vi "Halfband Filter.vi"() -> ()   [LabVIEW 2023]
doc: "Demonstrates how to use the DFD Halfband Design VI to design a halfband finite impulse response (FIR) filter.\n\nComplete the following steps to use this VI.\n1) Run the VI.\n2) Change the specifications and run this VI again.\n3) Observe the Coefficients and Magnitude Response graphs. Notice that the filter coefficients equal zero every other coefficient except for the middle coefficient."
uses:
  <vilib>/addons/Digital Filter Design/_Objects.llb/DFD Multirate Filtering Mode.ctl
  <vilib>/addons/Digital Filter Design/NI_DigFilterLicensed.lvlib
panel:
  out "Error Message":string
  in  "Method":u16(ring)=3 items=["Kaiser Window", "Dolph-Chebyshev Window", "Equi-Ripple", "Positive Equi-Ripple", "Max Flat"]
  in  "Filter Type":enum16{"Lowpass", "Highpass"}(ring)
  in  "Roll Off":dbl=0.1
  out "Magnitude Response":cluster{"f0":dbl, "df":dbl, "values":dbl[]}[](graph)
  out "Coefficients":dbl[](graph)
  in  "Stopband Attenuation [dB]":dbl=40.0 format="%.2f"
  # "Select Help>>Show Context Help and move the cursor over the VI icon for more information."
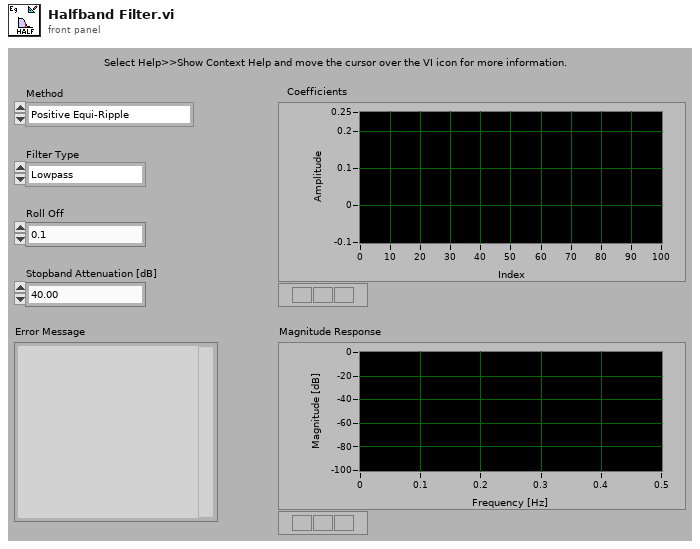
[diagram p1: front panel]
types:
  T1 = typedef "NI_DigFilterLicensed.lvlib/DFD Multirate Filtering Mode.ctl" = u16
  T2 = typedef "NI_DigFilterLicensed.lvlib/DFD Multirate Filter Obj.ctl" = cluster{"mMRate_Structure":enum16{"CIC", "FIR", "IIR", "Lattice"}, "mMRate_Mode":T3, "mMRate_Factor":i32, "mMRate_FIRParams":cluster{"mMRate_FIR_H":dbl[], "mMRate_FIR_IsNyquist?":bool, "mMRate_FIR_IsSymmetric?":bool}, "mMRate_CICParams":cluster{"mMRate_CIC_#Stage":i32, "mMRate_CIC_Lag":i32, "mMRate_CIC_Type":enum16{"Lowpass", "Highpass"}}, "mMRate_Order":i32, "mMRate_Version":string, "mMRate_Comments":string, "mMRate_RationalFactor":cluster{"mMRate_L":i32, "mMRate_M":i32}, "mMRate_Fs":dbl, "mMRate_Quantized?":bool, "mMRate_QFilterGain":dbl, "mMRate_CoefWl":i16, "mMRate_Scaling":cluster{"mMRate_ScaleByPowerOf2?":bool, "mMRate_ScaleType":T4}, "mMRate_InputWl":i16, "mMRate_OutputWl":i16, "mMRate_OutputMode":T5, "mMRate_MultMode":T6, "mMRate_BitPruning":bool, "mMRate_GainWl":i16, "mMRate_OutputFwl":i16, "mMRate_SumIwl":i16, "mMRate_InputIwl ":i16, "mMRate_SumWl":i16, "mMRate_CoefIwl":i16}
  T3 = typedef "NI_DigFilterLicensed.lvlib/DFD Multirate Mode.ctl" = i16
  T4 = typedef "NI_DigFilterLicensed.lvlib/DFD Coef Norm Type.ctl" = enum16{"No Norm", "Time Domain 1-Norm", "Time Domain 2-Norm", "Time Domain Inf-Norm"}
  T5 = typedef "NI_DigFilterLicensed.lvlib/DFD Round-off Mode.ctl" = enum16{"Nearest", "Truncation"}
  T6 = typedef "NI_DigFilterLicensed.lvlib/DFD FXP MRate Multiply Mode.ctl" = enum16{"Truncated", "Full"}
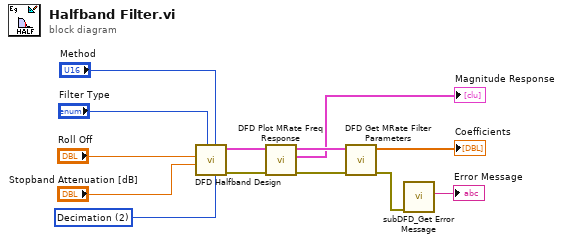
[diagram p0: block diagram]
diagram:
  w3 = T1 2 items=["No Rate Change", "Interpolation", "Decimation"] ("filtering mode")
  n1 = call <vilib>:"DFD Halfband Design.vi"("filtering mode"=w3, "method"="Method", "filter type"="Filter Type", "stopband attenuation [dB]"="Stopband Attenuation [dB]", "roll off"="Roll Off") -> ("error out"=w11:errorcluster, "multirate filter out"=w12:T2)  [unwired: 3 in, 2 out]
  n2 = call <vilib>:"DFD Plot MRate Freq Response.vi"("error in (no error)"=w11, "multirate filter in"=w12) -> ("error out"=w9:errorcluster, "magnitude response"=→"Magnitude Response":cluster{"f0":dbl, "df":dbl, "values":dbl[]}[], "multirate filter out"=w8:T2)  [unwired: 5 in, 2 out]
  n3 = call <vilib>:"DFD Get MRate Filter Parameters.vi"("error in (no error)"=w9, "multirate filter in"=w8) -> ("error out"=w1:errorcluster, "h(n)"=→"Coefficients":dbl[])  [unwired: 1 in, 7 out]
  n4 = call <vilib>:"subDFD_Get Error Message.vi"("error in (no error)"=w1) -> ("Error Message"=→"Error Message":string)  [unwired: 10 out]
